vi "Obtain ADC measurement.vi"(4 "index":i32, 6 "Expected Reading":dbl, 7 "DAC Channel Name":string) -> (1 "Aborted":bool, 3 "Reading":string)   [LabVIEW 2015]
panel:
  out "Tab Control":enum32{"Page 2", "Page 1"}(tab)
  in  "AbortButton":bool
  in  "Actual Reading":string
  in  "Done":bool
  # "Please enter the measured value for the ADC channel listed below \n(Use the attached picture to locate test point)"
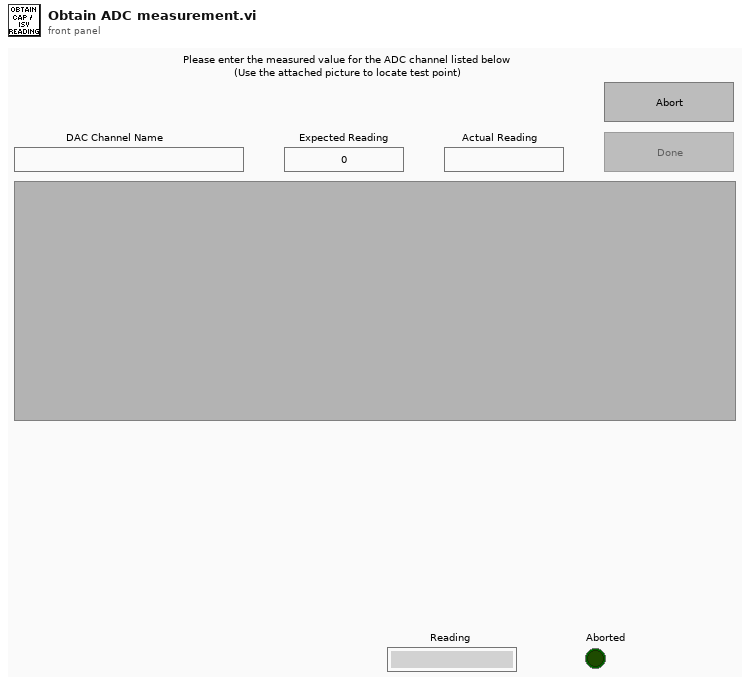
[diagram p1: front panel]
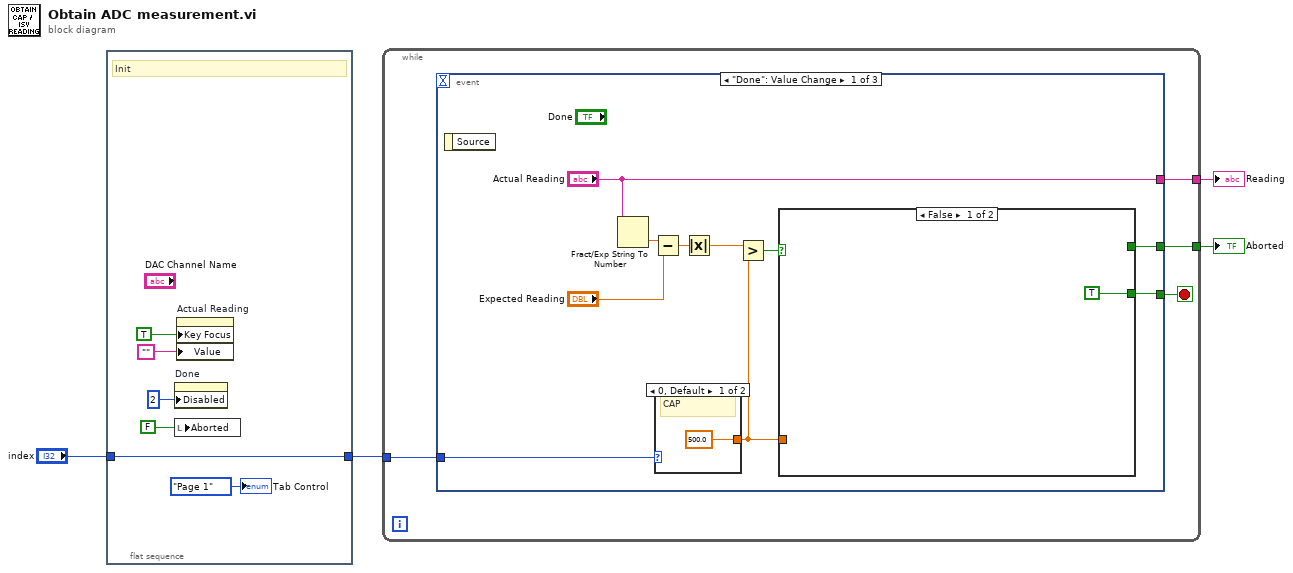
[diagram p0: block diagram]
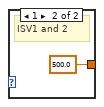
[diagram p2: hidden frame]
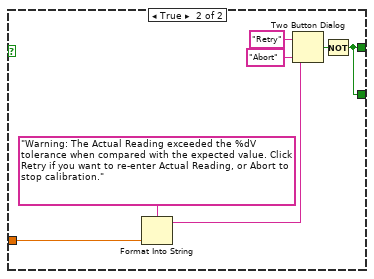
[diagram p3: hidden frame]
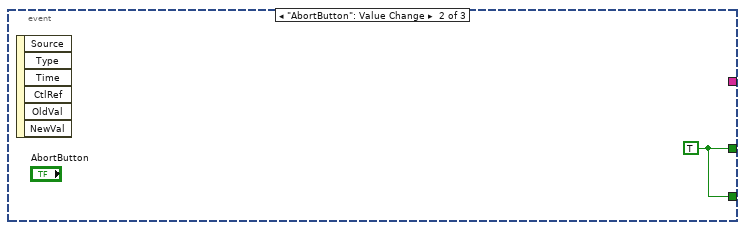
[diagram p4: hidden frame]
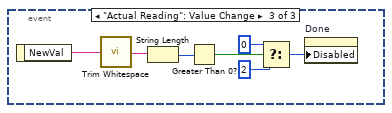
[diagram p5: hidden frame]
diagram:
  n1 = flat-sequence {
    tunnel: "index" -> [w6]
    tunnel: [w6] -> w3
    frame #0 {
      # "Init"
      n2 = property on="Done" class="Bool"("Disabled"=u8 2) -> ()  [unwired: 2 in, 2 out]
      n3 = local write "Aborted"(FALSE ("Aborted")) -> ()
      n4 = property on="Actual Reading" class="Str"("Key Focus"=TRUE, "Value"="") -> ()  [unwired: 2 in, 2 out]
      "Tab Control" <- enum32{"Page 2", "Page 1"}."Page 1" ("Tab Control")
    }
  }
  n5 = while {
    tunnel: w3 -> [w14]
    tunnel: [w13] -> w2
    tunnel: [w12] -> w1
    stop <- w11 stop-if-true
    n6 = event shown="[0] \"Done\": Value Change" {
      selector: _ -> [_ _ _]
      dyn-events: _ -> [_ _ _]
      timeout: _ -> [_ _ _]
      tunnel: w14 -> [w21 _ _]
      tunnel: ["Actual Reading" _ _] -> w13
      tunnel: [w16 w35 _] -> w12
      tunnel: [w15 w35 _] -> w11
      event "Done": Value Change {
        n7 = event-data() -> ()  [unwired: 2 out]
        n8 = Fract/Exp String To Number(string="Actual Reading") -> (number=w24:dbl)  [unwired: 4 out]
        n9 = Subtract(x=w24, y="Expected Reading") -> (x-y=w23:dbl)
        n10 = case shown="0, Default" w21 {
          tunnel: [500.0 ("Expected Reading") 500.0 ("Expected Reading")] -> w18
          frame 0, Default {
            # "CAP"
          }
          frame 1 {
            # "ISV1 and 2"
          }
        }
        n11 = Absolute Value(x=w23) -> (abs(x)=w20:dbl)
        n12 = Greater?(x=w20, y=w18) -> (0:w19:bool)
        n13 = case shown="False" w19 {
          tunnel: w18 -> [_ w32]
          tunnel: [_ w28] -> w16
          tunnel: [TRUE w28] -> w15
          frame False {
          }
          frame True {
            n14 = Format Into String(format string="Warning: The Actual Reading exceeded the %dV tolerance when compared with the expected value. Click Retry if you want to re-enter Actual Reading, or Abort to stop calibration.", w32) -> (resulting string=w30:string)  [unwired: 2 in, 1 out]
            n15 = Two Button Dialog(message=w30, 1:"Abort" ("F button name (\"Cancel\")"), 2:"Retry" ("T button name (\"OK\")")) -> (T button?=w29:bool)
            n16 = Not(x=w29) -> (.not. x?=w28:bool)
          }
        }
      }
      event "AbortButton": Value Change {
        w35 = TRUE ("Aborted")
        n17 = event-data() -> ()  [unwired: 7 out]
      }
      event "Actual Reading": Value Change {
        n18 = event-data() -> ("NewVal"=w37:string)  [unwired: 1 out]
        n19 = call <vilib>:"Trim Whitespace.vi"("string"=w37) -> ("trimmed string"=w42:string)  [unwired: 1 in]
        n20 = String Length(string=w42) -> (length=w41:i32)
        n21 = Greater Than 0?(x=w41) -> (x > 0?=w36:bool)
        n22 = Select(t=u8 0, s=w36, f=u8 2 ("Disabled")) -> (s? t:f=w38:u8)
        n23 = property on="Done" class="Bool"("Disabled"=w38) -> ()  [unwired: 2 in, 2 out]
      }
    }
  }
  "Reading" <- w2
  "Aborted" <- w1
